vi "ABR3-Save Data.vi"(0 "Runtime":T3={"Ceiling"=0.0, "Threshold"=0.0, "Crossed?"=FALSE, "Step"=0, "Stop"=0, "Avgs"=0, "Level"=0.0, "AI Npts"=0, "Doubled?"=FALSE, "Gain"=0.0, "NWindowPts"=0, "dt"=0.0, "Cal"=path "", "Freq"=0.0, "AO Channels"=[], "AltPol"=FALSE, "AO Npts"=0, "AO Fs"=0.0, "Start"=0, "Stop max"=0, "Ear"=enum."Right", "Waveform"=enum."TONE PIP", "RepRate"=0.0, "CAP or ABR"=1, "LMasker"=0.0, "SeqVar"=enum."Signal Level", "Reps/buffer"=0, "Avg Mode"=enum."Neural/CM", "Wav"=path "", "Order"=enum."Sequential", "Levels"=[], "ControlVal"=0.0, "innerIndex"=0, "indexStep"=0} {"CAP or ABR" items=["CAP", "ABR"]}, 1 "State (in)":T7, 9 "Aborted?":bool, 11 "error in (no error)":errorcluster, 12 "Notes":string, 13 "Analysis":T1) -> (3 "State (out)":T7, 4 "Run #":i16, 6 "Datafile path":path, 10 "Saved?":bool, 15 "error out":errorcluster)   [LabVIEW 2020]
uses:
  CFTS Main Panel SubVIs/CFTS-Experiment State.ctl
  TypeDefs/ABR3-Runtime Data.ctl
  epl-vi-lib/Utility VIs/Type Defs/Left-Right ring.ctl
  TypeDefs/ABR-Waveform Enum.ctl
  TypeDefs/ABR3-Seq Var Enum.ctl
  TypeDefs/ABR3-Analysis State.ctl
  Threshold Estimation VIs/ABR3-Threshold Estimation Result.ctl
  epl-vi-lib/Utility VIs/File IO VIs/Configuration File Wrapper VIs/Config-Read Key (string).vi
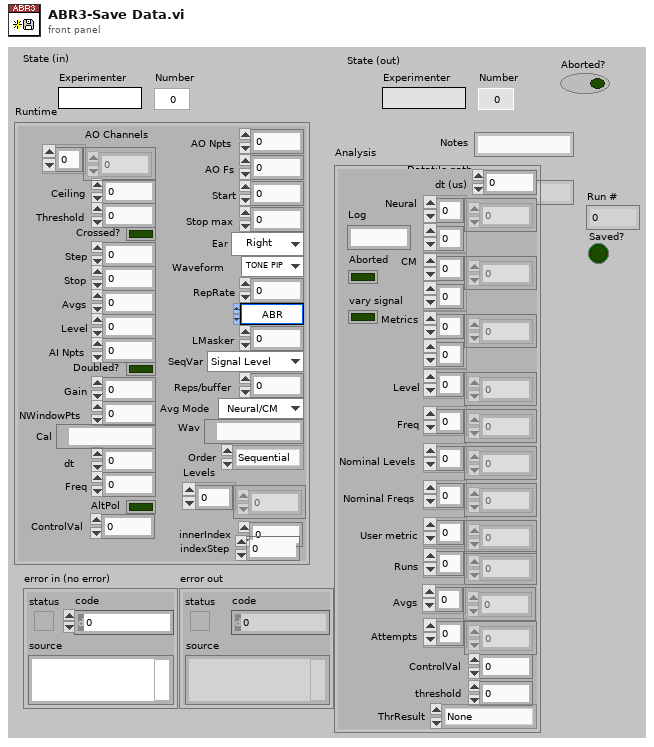
[diagram p1: front panel]
types:
  T1 = typedef "ABR3-Analysis State.ctl" = cluster{"dt (us)":dbl, "Neural":dbl[][], "CM":dbl[][], "Metrics":dbl[][], "Level":dbl[], "Freq":dbl[], "Nominal Levels":dbl[], "Nominal Freqs":dbl[], "User metric":dbl[], "Runs":i32[], "Avgs":i32[], "Attempts":i32[], "Log":string, "Aborted":bool, "ControlVal":dbl, "threshold":dbl, "vary signal":bool, "ThrResult":T2}
  T2 = typedef "ABR3-Threshold Estimation Result.ctl" = enum16{"None", "Power", "Sigmoid", "Power (noisy)", "Suprathreshold", "Invalid"}
  T3 = typedef "ABR3-Runtime Data.ctl" = cluster{"Ceiling":dbl, "Threshold":dbl, "Crossed?":bool, "Step":i32, "Stop":i32, "Avgs":i32, "Level":dbl, "AI Npts":i32, "Doubled?":bool, "Gain":dbl, "NWindowPts":i32, "dt":dbl, "Cal":path, "Freq":dbl, "AO Channels":i32[], "AltPol":bool, "AO Npts":i32, "AO Fs":dbl, "Start":i32, "Stop max":i32, "Ear":T4, "Waveform":T5, "RepRate":dbl, "CAP or ABR":u16, "LMasker":dbl, "SeqVar":T6, "Reps/buffer":i32, "Avg Mode":enum16{"Neural/CM", "ANOW"}, "Wav":path, "Order":enum16{"Sequential", "Random"}, "Levels":dbl[], "ControlVal":dbl, "innerIndex":i32, "indexStep":i32}
  T4 = typedef "Left-Right ring.ctl" = enum16{"Right", "Left"}
  T5 = typedef "ABR-Waveform Enum.ctl" = enum16{"TONE PIP", "CLICK", "FILE", "CHIRP", "NOISE", "VERHULST"}
  T6 = typedef "ABR3-Seq Var Enum.ctl" = enum16{"Signal Level", "Masker Level"}
  T7 = typedef "CFTS-Experiment State.ctl" = cluster{"Experimenter":string, "Number":u32, "Right":string, "Left":string, "Data Folder":path, "State File":path, "Version Info":string, "End Exposure Time":dbl, "Exposure Duration":string, "Run #":cluster{"CAP":i16, "ABR":i16, "DP":i16, "VsEP":i16, "MeasSeq":i16, "SubSeq":i16, "SFOAE":i16}}
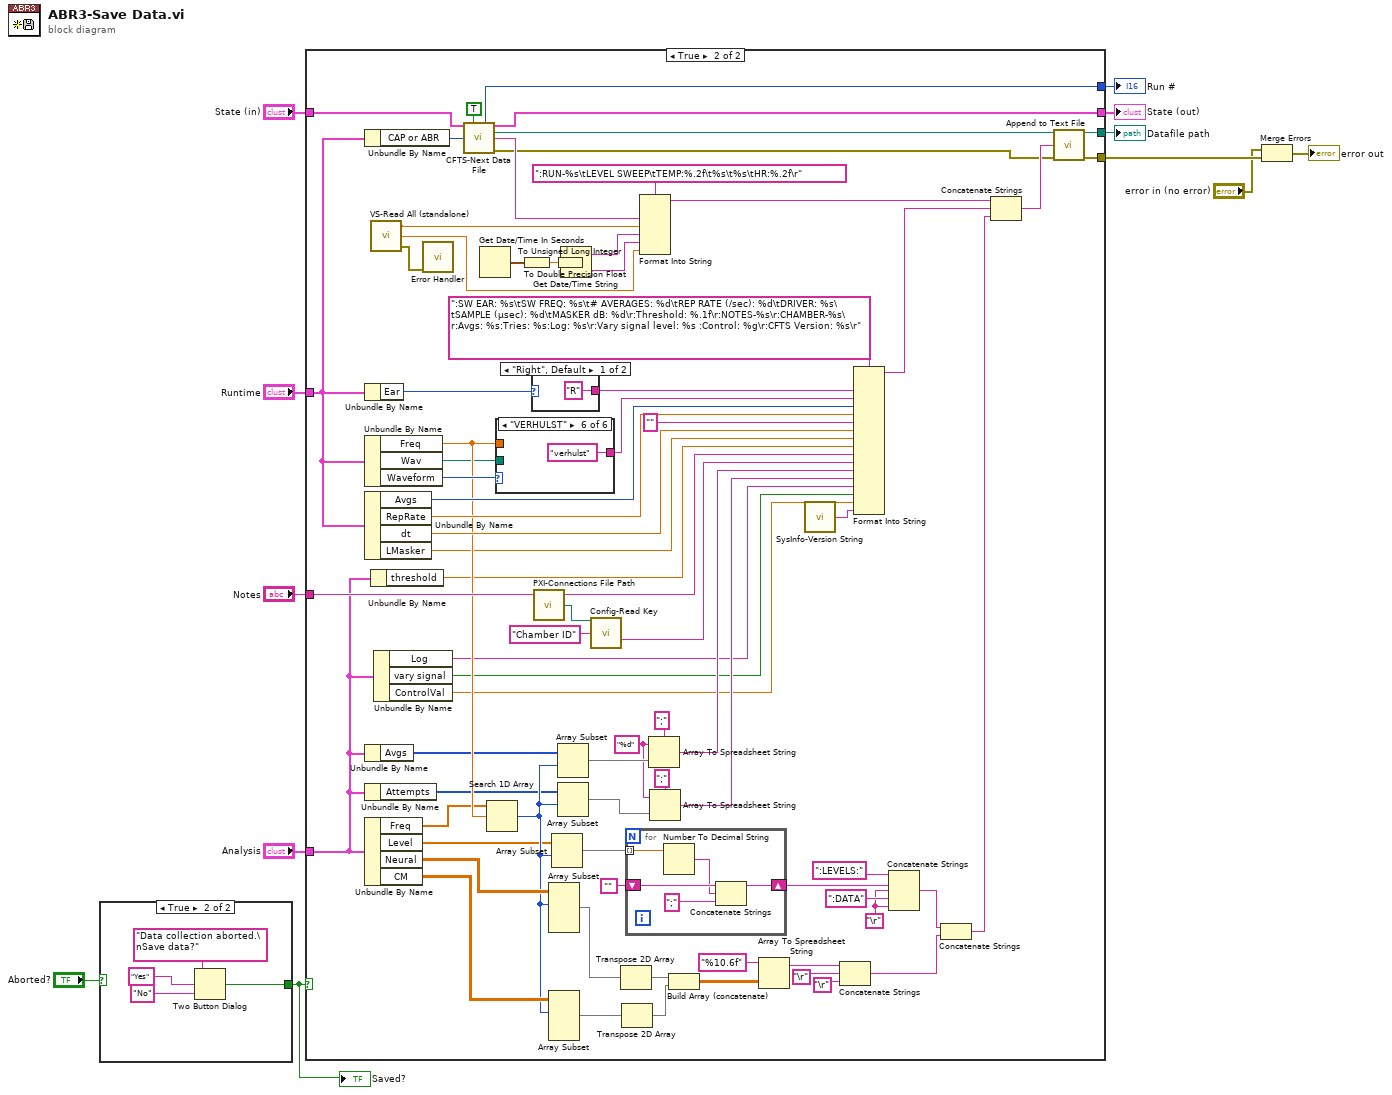
[diagram p0: block diagram]
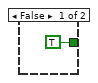
[diagram p2: hidden frame]
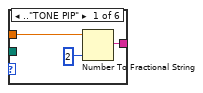
[diagram p4: hidden frame]
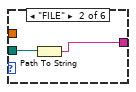
[diagram p5: hidden frame]
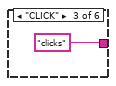
[diagram p6: hidden frame]
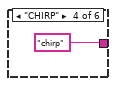
[diagram p7: hidden frame]
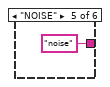
[diagram p8: hidden frame]
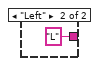
[diagram p9: hidden frame]
diagram:
  n1 = case shown="True" "Aborted?" {
    tunnel: [TRUE ("T button?") w14] -> w1
    frame False {
    }
    frame True {
      n2 = Two Button Dialog(message="Data collection aborted.\nSave data?", 1:"No" ("F button name (\"Cancel\")"), 2:"Yes" ("T button name (\"OK\")")) -> (T button?=w14:bool)
    }
  }
  "Saved?" <- w1
  n3 = case shown="True" w1 {
    tunnel: "State (in)" -> [w18 w95]
    tunnel: [w18 w94] -> w11
    tunnel: [_ w81] -> w10
    tunnel: "Runtime" -> [_ w27]
    tunnel: "Notes" -> [_ w71]
    tunnel: [_ w70] -> w6
    tunnel: "Analysis" -> [_ w20]
    tunnel: [_ w48] -> w4
    frame False {
    }
    frame True {
      w33 = "%d" ("format string")
      w64 = "\r"
      n4 = Unbundle By Name(w27) -> ("CAP or ABR"=w69:u16)
      n5 = Unbundle By Name(w27) -> ("Ear"=w79:T4)
      n6 = Unbundle By Name(w27) -> ("Freq"=w53:dbl, "Wav"=w41:path, "Waveform"=w76:T5)
      n7 = Unbundle By Name(w27) -> ("Avgs"=w75:i32, "RepRate"=w74:dbl, "dt"=w72:dbl, "LMasker"=w45:dbl)
      n8 = Unbundle By Name(w20) -> ("Avgs"=w39:i32[])
      n9 = Unbundle By Name(w20) -> ("Attempts"=w35:i32[])
      n10 = Unbundle By Name(w20) -> ("Freq"=w46:dbl[], "Level"=w26:dbl[], "Neural"=w52:dbl[][], "CM"=w50:dbl[][])
      n11 = call "VS-Read All (standalone).vi"() -> ("error out"=w43:errorcluster, "Heart Rate (bpm)"=w42:dbl, "Temperature (C)"=w44:dbl)  [unwired: 3 in]
      n12 = Unbundle By Name(w20) -> ("threshold"=w19:dbl)
      n13 = Unbundle By Name(w20) -> ("Log"=w29:string, "vary signal"=w25:bool, "ControlVal"=w24:dbl)
      n14 = call "Error Handler.vi"("error in (no error)"=w43) -> ()  [unwired: 13 in, 2 out]
      n15 = call "CFTS-Next Data File.vi"("Expt State"=w95, "Allow overwrite"=TRUE, "Data Type"=w69) -> ("Run #"=w70:i16, "Expt State out"=w94:T7, "Datafile path"=w84:path, "run #"=w87:string, "error out"=w82:errorcluster)  [unwired: 8 in]
      n16 = Get Date/Time In Seconds() -> (seconds since 1Jan1904=w91:timestamp)
      n17 = Search 1D Array(1D array=w46, element=w53) -> (index of element=w36:i32)  [unwired: 1 in]
      n18 = case shown="\"VERHULST\"" w76 {
        tunnel: [w102 w104 "clicks" "chirp" "noise" "verhulst"] -> w77
        tunnel: w53 -> [w103 _ _ _ _ _]
        tunnel: w41 -> [_ w105 _ _ _ _]
        frame .."TONE PIP" {
          n19 = Number To Fractional String(number=w103, precision (6)=2) -> (F-format string=w102:string)  [unwired: 2 in]
        }
        frame "FILE" {
          n20 = Path To String(path=w105) -> (string=w104:string)
        }
        frame "CLICK" {
        }
        frame "CHIRP" {
        }
        frame "NOISE" {
        }
        frame "VERHULST" {
        }
      }
      n21 = To Double Precision Float(number=w91) -> (double precision float=w90:dbl)
      n22 = case shown="\"Right\", Default" w79 {
        tunnel: ["R" "L"] -> w78
        frame "Right", Default {
        }
        frame "Left" {
        }
      }
      n23 = call "PXI-Connections File Path.vi"() -> ("Path"=w22:path)  [unwired: 1 in]
      n24 = Array Subset(array=w52, index (row)=w36) -> (w51:dbl[][])  [unwired: 3 in]
      n25 = Array Subset(array=w50, index (row)=w36) -> (w49:dbl[][])  [unwired: 3 in]
      n26 = Array Subset(array=w26, index=w36) -> (w47:dbl[])  [unwired: 1 in]
      n27 = To Unsigned Long Integer(number=w90) -> (unsigned 32bit integer=w89:u32)
      n28 = Array Subset(array=w39, index=w36) -> (w38:i32[])  [unwired: 1 in]
      n29 = Array Subset(array=w35, index=w36) -> (w32:i32[])  [unwired: 1 in]
      n30 = Get Date/Time String(seconds (now)=w89) -> (date string=w92:string, time string=w93:string)  [unwired: 2 in]
      n31 = call-poly "Config-Read Key.vi"("configuration file path"=w22, "key"="Chamber ID" ("string")) -> ("value"=w21:string)  [unwired: 10 in, 3 out]
      n32 = Transpose 2D Array(2D array=w51) -> (transposed array=w58:dbl[][])
      n33 = Transpose 2D Array(2D array=w49) -> (transposed array=w57:dbl[][])
      n34 = for {
        shift-right: [w97] -> w65
        shift-left: "" -> [w100]
        tunnel: w47 -> [w96] mode=indexing
        n35 = Number To Decimal String(number=w96) -> (decimal integer string=w99:string)  [unwired: 1 in]
        n36 = Concatenate Strings(w100, w99, ";") -> (w97:string)
      }
      n37 = Format Into String(format string=":RUN-%s\tLEVEL SWEEP\tTEMP:%.2f\t%s\t%s\tHR:%.2f\r", w87, w44, w92, w93, w42) -> (resulting string=w86:string)  [unwired: 2 in, 1 out]
      n38 = Array To Spreadsheet String(delimiter (Tab)=";", array=w38, 3:w33) -> (spreadsheet string=w37:string)
      n39 = Array To Spreadsheet String(delimiter (Tab)=";", array=w32, 3:w33) -> (spreadsheet string=w31:string)
      n40 = Build Array (concatenate)(w58, w57) -> (w56:dbl[][])
      n41 = Array To Spreadsheet String(array=w56, 3:"%10.6f") -> (spreadsheet string=w61:string)  [unwired: 1 in]
      n42 = call "SysInfo-Version String.vi"() -> ("Version String"=w30:string)  [unwired: 1 in]
      n43 = Concatenate Strings(w61, "\r", "\r") -> (w55:string)
      n44 = Format Into String(format string=":SW EAR: %s\tSW FREQ: %s\t# AVERAGES: %d\tREP RATE (/sec): %d\tDRIVER: %s\tSAMPLE (µsec): %d\tMASKER dB: %d\r:Threshold: %.1f\r:NOTES-%s\r:CHAMBER-%s\r:Avgs: %s:Tries: %s:Log: %s\r:Vary signal level: %s :Control: %g\r:CFTS Version: %s\r", w78, w77, w75, w74, "" ("input 5"), w72, w45, w19, w71, w21, w37, w31, w29, w25, w24, w30) -> (resulting string=w80:string)  [unwired: 2 in, 1 out]
      n45 = Concatenate Strings(":LEVELS:", w65, w64, ":DATA", w64) -> (w63:string)
      n46 = Concatenate Strings(w63, w55) -> (w54:string)
      n47 = Concatenate Strings(w86, w80, w54) -> (w83:string)
      n48 = call "Append to Text File.vi"("file path"=w84, "text"=w83, "error in (no error)"=w82) -> ("file path out"=w81:path, "error out"=w48:errorcluster)  [unwired: 11 in]
    }
  }
  "State (out)" <- w11
  "Datafile path" <- w10
  "Run #" <- w6
  n49 = Merge Errors("error in (no error)", w4) -> (→"error out":errorcluster)
